vi "GetHelp.vi"(11 "Test in":refnum<class "Test.lvclass">) -> (2 "Help":string, 3 "Test out":refnum<class "Test.lvclass">)   [LabVIEW 2014, in "Test.lvclass"]
uses:
  Test.lvclass
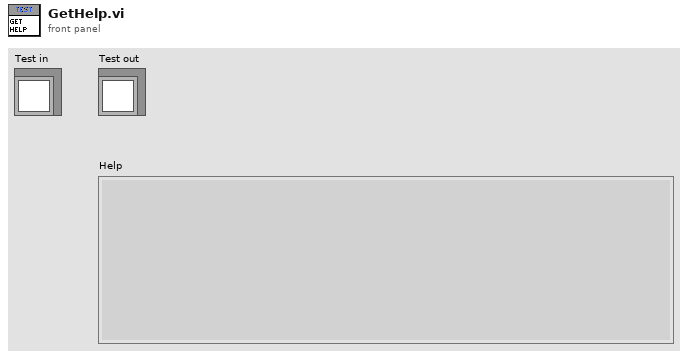
[diagram p1: front panel]
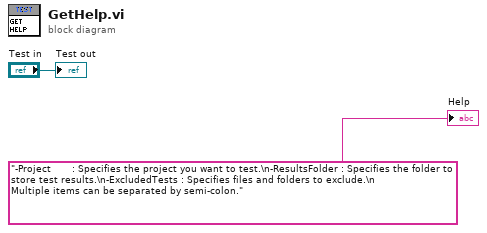
[diagram p0: block diagram]
diagram:
  "Test out" <- "Test in"
  "Help" <- "-Project       : Specifies the project you want to test.\n-ResultsFolder : Specifies the folder to store test results.\n-ExcludedTests : Specifies files and folders to exclude.\n                 Multiple items can be separated by semi-colon." ("Help")
